vi "MainConvertiMisure_INPUT.vi"(6 "SET Q A ZERO":T1, 8 "canale--sensore":string[][](array[string]), 9 "Assoc_input_sensori":string[][](array[string]), 10 "Array Misure Input":dbl[](array[numeric]), 11 "Caratteristiche canali Caricate":string[][](array[string])) -> (2 "Array Misure/Unità OUT":T2[](array[typedef]))   [LabVIEW 2019]
uses:
  <vilib>/Analysis/6fits.llb/Curve Fitting Criteria.ctl
  <vilib>/Analysis/polynomials.llb/Scalar Polynomial Evaluation (DBL).vi
  <vilib>/Analysis/NI_AALPro.lvlib
  <vilib>/gmath/NI_Gmath.lvlib
panel:
  in  "Cluster Misura / Unità":T2
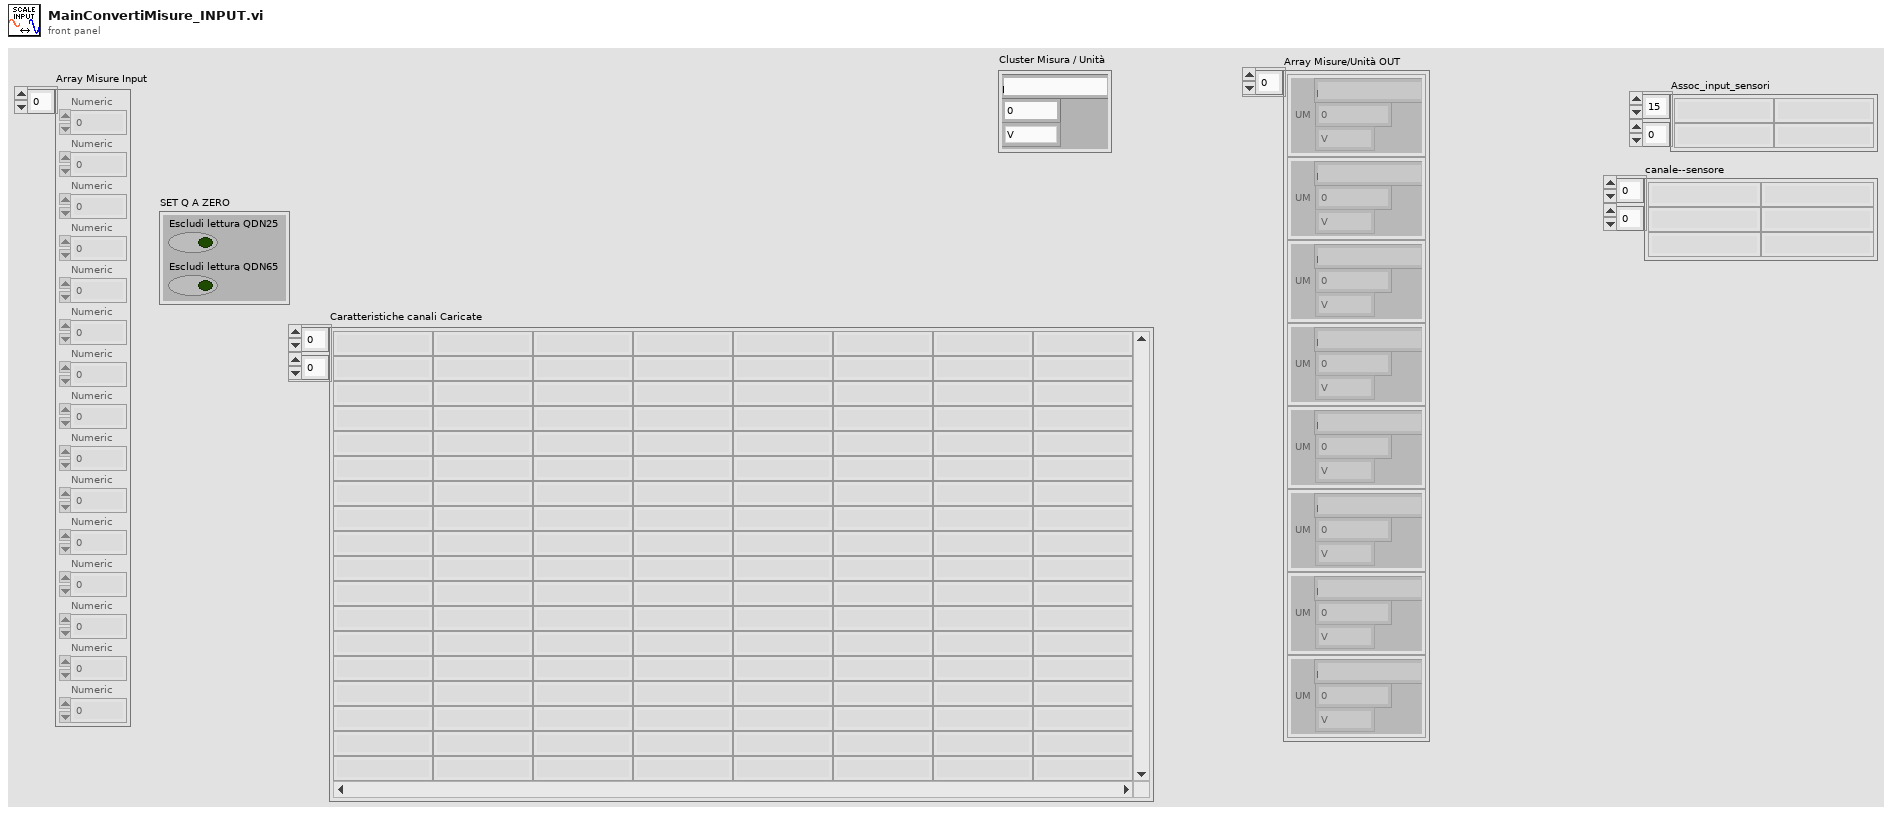
[diagram p1: front panel]
types:
  T1 = cluster{"Escludi lettura QDN25":bool, "Escludi lettura QDN65":bool}
  T2 = typedef "ClusterMisura_e_Unità_INPUT.ctl" = cluster{"Misura":dbl, "UM":T3, "Descrizione":string}
  T3 = typedef "UnitàMisura.ctl" = enum16{"V", "mA", "Bar", "RPM", "m3/s", "m3/min", "m3/h", "l/s", "l/min", "in3/min", "ft3/min", "gpm", "igpm", "igph", "%", "°C", "m", "Nm", "A"}
  T4 = cluster{"impostazioni conversione":string[], "um":i32}
  T5 = cluster{"ordine polinomiale":i32, "X":dbl[], "Y":dbl[]}
  T6 = typedef "NI_AALPro.lvlib/Curve Fitting Criteria.ctl" = u16
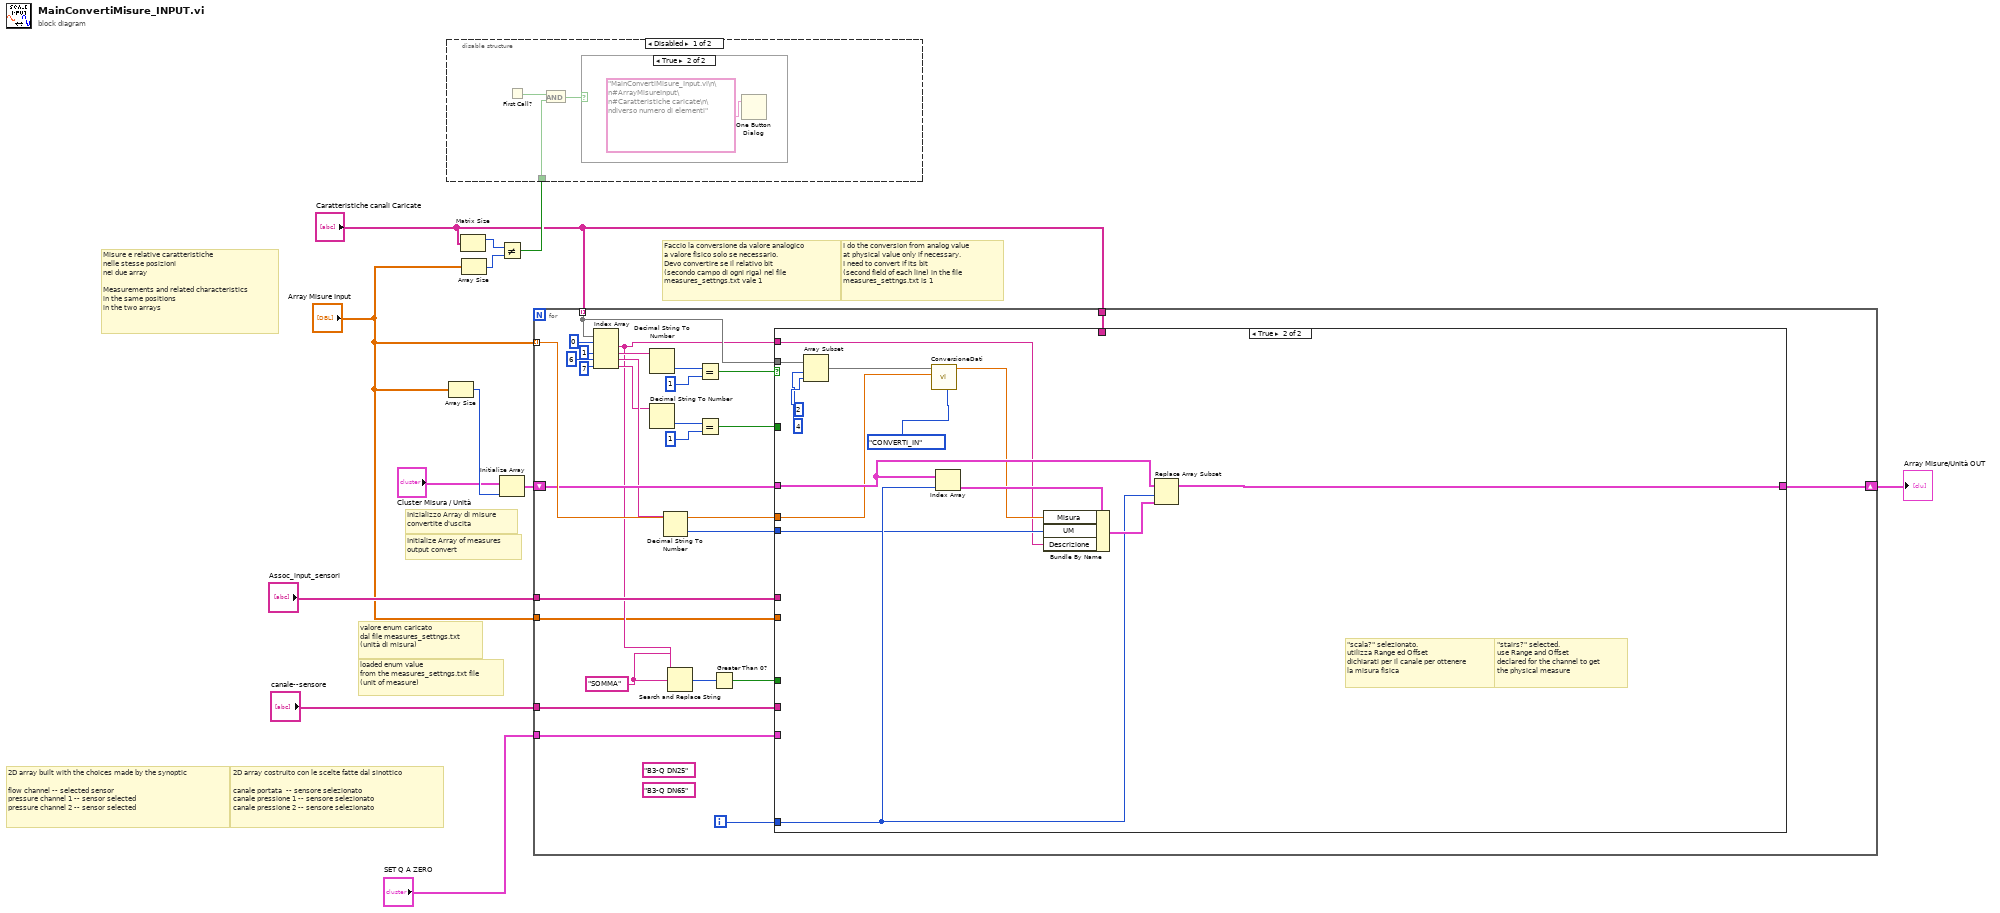
[diagram p0: block diagram]
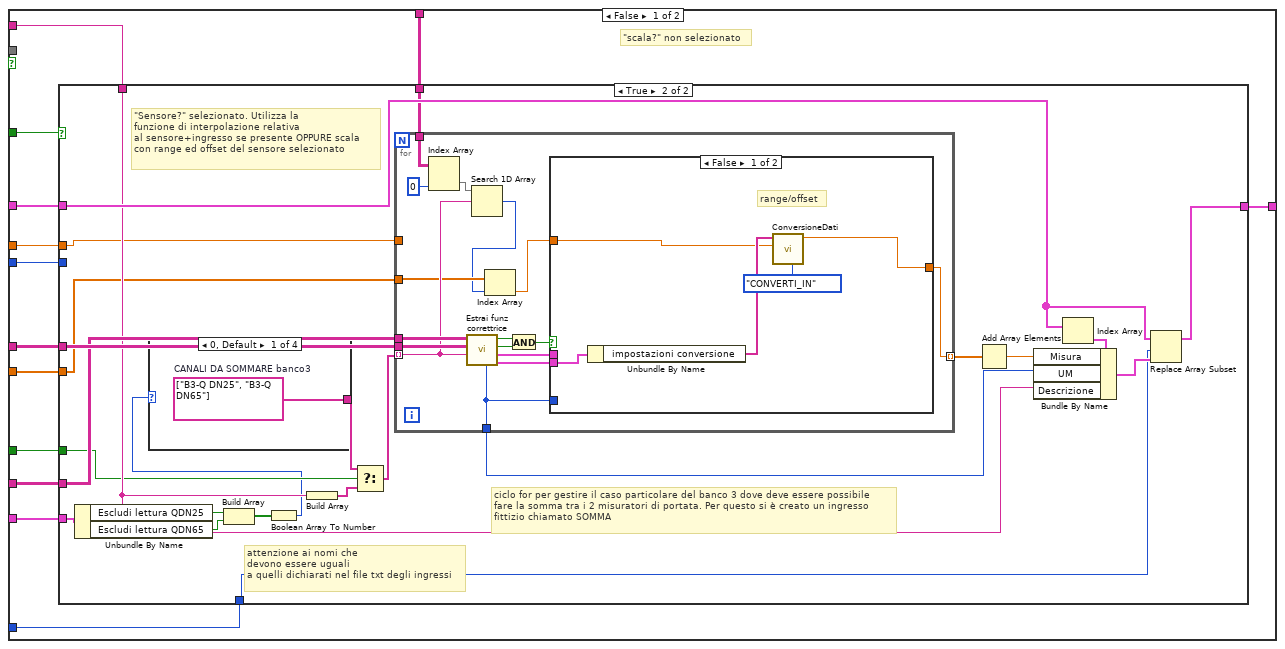
[diagram p4: hidden frame]
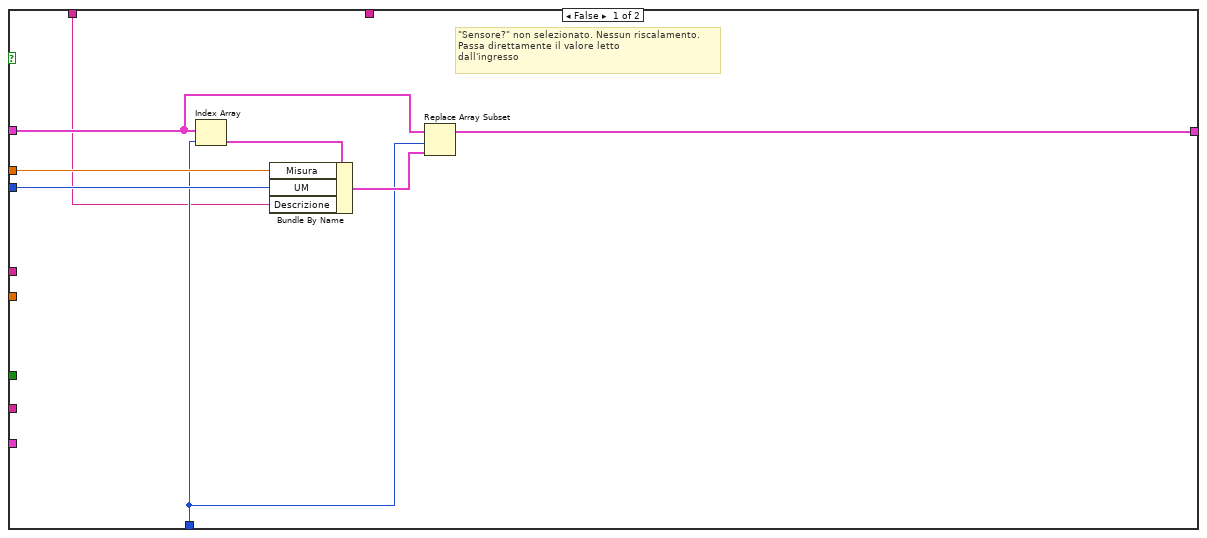
[diagram p5: hidden frame]
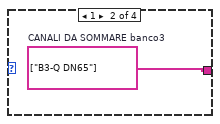
[diagram p6: hidden frame]
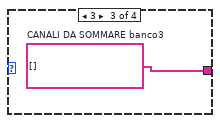
[diagram p7: hidden frame]
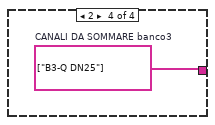
[diagram p8: hidden frame]
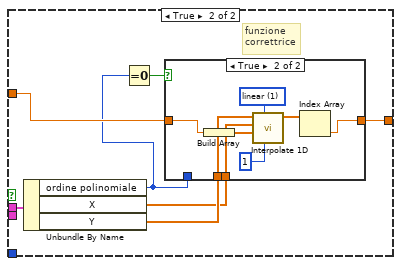
[diagram p9: hidden frame]
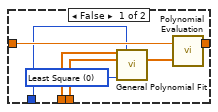
[diagram p10: hidden frame]
diagram:
  # "valore enum caricato\ndal file measures_settngs.txt \n(unità di misura)"
  # "loaded enum value\nfrom the measures_settngs.txt file\n(unit of measure)"
  # "Initialize Array of measures\noutput convert"
  # "2D array built with the choices made by the synoptic\n\nflow channel -- selected sensor\npressure channel 1 -- sensor selected\npressure channel 2 -- sensor selected"
  # "I do the conversion from analog value\nat physical value only if necessary.\nI need to convert if its bit\n(second field of each line) in the file\nmeasures_settngs.txt is 1"
  # "2D array costruito con le scelte fatte dal sinottico\n\ncanale portata  -- sensore selezionato\ncanale pressione 1 -- sensore selezionato\ncanale pressione 2 -- sensore selezionato"
  # "Faccio la conversione da valore analogico\na valore fisico solo se necessario. \nDevo convertire se il relativo bit \n(secondo campo di ogni riga) nel file \nmeasures_settngs.txt vale 1"
  # "Misure e relative caratteristiche\nnelle stesse posizioni\nnei due array\n\nMeasurements and related characteristics\nin the same positions\nin the two arrays"
  # "Inizializzo Array di misure \nconvertite d'uscita"
  n1 = Array Size(array="Array Misure Input") -> (size(s)=w12:i32)
  n2 = Matrix Size(0:"Caratteristiche canali Caricate") -> (1:w8:i32)  [unwired: 1 out]
  n3 = Array Size(array="Array Misure Input") -> (size(s)=w7:i32)
  n4 = Not Equal?(x=w8, y=w7) -> (x != y?=w6:bool)
  n5 = disable-structure shown="Disabled" {
    disable-tunnel: w6 -> [w14 _]
    frame Disabled {
      n6 = First Call?() -> (First Call?: T/F=w15:bool)
      n7 = And(x=w15, y=w14) -> (x .and. y?=w13:bool)
      n8 = case shown="True" w13 {
        frame False {
        }
        frame True {
          n9 = One Button Dialog(message="MainConvertiMisure_Input.vi\n\n#ArrayMisureInput\n#Caratteristiche caricate\n\ndiverso numero di elementi") -> ()  [unwired: 1 in, 1 out]
        }
      }
    }
    frame Enabled {
    }
  }
  n10 = Initialize Array("Cluster Misura / Unità", w12) -> (w11:T2[])
  n11 = for {
    tunnel: "Array Misure Input" -> [w39] mode=indexing
    tunnel: "Caratteristiche canali Caricate" -> [w33] mode=indexing
    shift-right: [w34] -> w9
    shift-left: w11 -> [w38]
    tunnel: "Assoc_input_sensori" -> [w25]
    tunnel: "canale--sensore" -> [w24]
    tunnel: "Array Misure Input" -> [w19]
    tunnel: "Caratteristiche canali Caricate" -> [w18]
    tunnel: "SET Q A ZERO" -> [w17]
    i -> [w32]
    (unwired) "B3-Q DN65"
    (unwired) "B3-Q DN25"
    w23 = "SOMMA" ("search string")
    n12 = Index Array(array=w33, index #1=0 ("index"), index #2=1 ("index"), index #3=6 ("index"), index #4=7 ("index")) -> (element #1=w21:string, element #2=w43:string, element #3=w36:string, element #4=w27:string)
    n13 = Decimal String To Number(string=w43) -> (number=w42:i32)  [unwired: 2 in, 1 out]
    n14 = Decimal String To Number(string=w27) -> (number=w28:i32)  [unwired: 2 in, 1 out]
    n15 = Decimal String To Number(string=w36) -> (number=w35:i32)  [unwired: 2 in, 1 out]
    n16 = Search and Replace String(input string=w21, search string=w23, replace string=w23) -> (number of replacements=w22:i32)  [unwired: 5 in, 3 out]
    n17 = Equal?(x=w42, y=1) -> (x = y?=w40:bool)
    n18 = Equal?(x=w28, y=1) -> (x = y?=w26:bool)
    n19 = Greater Than 0?(x=w22) -> (x > 0?=w20:bool)
    n20 = case shown="True" w40 {
      tunnel: w39 -> [w57 w141]
      tunnel: w38 -> [w55 w146]
      tunnel: w32 -> [w54 w148]
      tunnel: w35 -> [w56 w144]
      tunnel: [w53 w145] -> w34
      tunnel: w33 -> [_ w143]
      tunnel: w21 -> [w49 w136]
      tunnel: w26 -> [w52 _]
      tunnel: w25 -> [w51 _]
      tunnel: w24 -> [w50 _]
      tunnel: w20 -> [w48 _]
      tunnel: w19 -> [w47 _]
      tunnel: w18 -> [w46 _]
      tunnel: w17 -> [w45 _]
      frame False {
        # "\"scala?\" non selezionato"
        n21 = case shown="True" w52 {
          tunnel: w57 -> [w64 w78]
          tunnel: w56 -> [w63 _]
          tunnel: w55 -> [w61 w83]
          tunnel: w54 -> [w60 w84]
          tunnel: [w59 w82] -> w53
          tunnel: w49 -> [w58 w80]
          tunnel: w51 -> [_ w88]
          tunnel: w50 -> [_ w87]
          tunnel: w48 -> [_ w73]
          tunnel: w47 -> [_ w72]
          tunnel: w46 -> [_ w71]
          tunnel: w45 -> [_ w70]
          frame False {
            # "\"Sensore?\" non selezionato. Nessun riscalamento.\nPassa direttamente il valore letto\ndall'ingresso"
            n22 = Index Array(array=w61, index=w60) -> (element=w65:T2)
            n23 = Bundle By Name(cluster=w65, "Misura"=w64, "UM"=w63, "Descrizione"=w58) -> (w62:T2)
            n24 = Replace Array Subset(array=w61, new element=w62, index=w60) -> (w59:T2[])
          }
          frame True {
            # "ciclo for per gestire il caso particolare del banco 3 dove deve essere possibile\nfare la somma tra i 2 misuratori di portata. Per questo si è creato un ingresso\nfittizio chiamato SOMMA"
            # "attenzione ai nomi che \ndevono essere uguali\na quelli dichiarati nel file txt degli ingressi"
            # "\"Sensore?\" selezionato. Utilizza la\nfunzione di interpolazione relativa\nal sensore+ingresso se presente OPPURE scala \ncon range ed offset del sensore selezionato"
            n25 = Unbundle By Name(w70) -> ("Escludi lettura QDN25"=w69:bool, "Escludi lettura QDN65"=w68:bool)
            n26 = Build Array(w69, w68) -> (w67:bool[])
            n27 = Boolean Array To Number(Boolean array=w67) -> (number=w66:u32)
            n28 = case shown="0, Default" w66 {
              tunnel: [w89 w90 w91 w92] -> w76
              frame 0, Default {
                w89 = string[] ["B3-Q DN25", "B3-Q DN65"]  # CANALI DA SOMMARE banco3
              }
              frame 1 {
                w90 = string[] ["B3-Q DN65"]  # CANALI DA SOMMARE banco3
              }
              frame 3 {
                w91 = string[] []  # CANALI DA SOMMARE banco3
              }
              frame 2 {
                w92 = string[] ["B3-Q DN25"]  # CANALI DA SOMMARE banco3
              }
            }
            n29 = Build Array(w80) -> (w75:string[])
            n30 = Select(t=w76, s=w73, f=w75) -> (s? t:f=w74:string[])
            n31 = for {
              tunnel: w88 -> [w108]
              tunnel: w87 -> [w107]
              tunnel: [w101] -> w81
              tunnel: [w100] -> w79 mode=indexing
              tunnel: w78 -> [_]
              tunnel: w74 -> [w96] mode=indexing
              tunnel: w72 -> [w95]
              tunnel: w71 -> [w99]
              n32 = Index Array(array=w99, index (col)=0 ("disabled index (col)")) -> (element=w97:string[])  [unwired: 1 in]
              n33 = call "Estrai funz correttrice.vi"("nome canale"=w96, "Assoc_input_sensori"=w108, "canale--sensore"=w107) -> ("conv. con range offset"=w104:T4, "INTERPOLAZIONE SETTINGS"=w105:T5, "USA FUNZ CORR"=w102:bool, "FUNZ CORR PRESENTE"=w103:bool, "um"=w101:i32)  [unwired: 4 in]
              n34 = Search 1D Array(1D array=w97, element=w96) -> (index of element=w94:i32)  [unwired: 1 in]
              n35 = Index Array(array=w95, index=w94) -> (element=w93:dbl)
              n36 = And(x=w103, y=w102) -> (x .and. y?=w106:bool)
              n37 = case shown="False" w106 {
                tunnel: w105 -> [_ w120]
                tunnel: w93 -> [w110 w117]
                tunnel: w104 -> [w112 _]
                tunnel: w101 -> [_ _]
                tunnel: [w109 w116] -> w100
                frame False {
                  # "range/offset"
                  n38 = Unbundle By Name(w112) -> ("impostazioni conversione"=w111:string[])
                  n39 = call "ConversioneDati.vi"("Stato Conversione"=enum16{"CONVERTI_IN", "CONVERTI_OUT"}."CONVERTI_IN", "Data"=w110, "Impostazioni Conversione"=w111) -> ("Dato Convertito"=w109:dbl)  [unwired: 8 in]
                }
                frame True {
                  # "funzione\ncorrettrice"
                  n40 = Unbundle By Name(w120) -> ("ordine polinomiale"=w114:i32, "X"=w118:dbl[], "Y"=w119:dbl[])
                  n41 = Equal To 0?(x=w114) -> (x = 0?=w115:bool)
                  n42 = case shown="True" w115 {
                    tunnel: w119 -> [w126 w134]
                    tunnel: w118 -> [w125 w135]
                    tunnel: w117 -> [w123 w129]
                    tunnel: [w122 w130] -> w116
                    tunnel: w114 -> [w121 _]
                    frame False {
                      w127 = T6 0 items=["Least Square", "Least Absolute Residual", "Bisquare"] ("method")
                      n43 = call <vilib>:"General Polynomial Fit.vi"("Y"=w126, "polynomial order"=w121, "X"=w125, "method"=w127) -> ("Polynomial Coefficients"=w124:dbl[])  [unwired: 8 in, 3 out]
                      n44 = call-poly <vilib>:"Polynomial Evaluation.vi"("P(x)"=w124, "a"=w123) -> ("P(a)"=w122:dbl)  [unwired: 1 out]
                    }
                    frame True {
                      w133 = 1 items=["nearest", "linear", "spline", "cubic Hermite", "Lagrange"] ("method")
                      n45 = Build Array(w129) -> (w128:dbl[])
                      n46 = call <vilib>:"Interpolate 1D.vi"("ntimes"=1, "method"=w133, "xi"=w128, "X"=w135, "Y"=w134) -> ("yi"=w131:dbl[])  [unwired: 4 in, 2 out]
                      n47 = Index Array(array=w131) -> (element=w130:dbl)  [unwired: 1 in]
                    }
                  }
                }
              }
            }
            n48 = Add Array Elements(numeric array=w79) -> (sum=w77:dbl)
            n49 = Index Array(array=w83) -> (element=w86:T2)  [unwired: 1 in]
            n50 = Bundle By Name(cluster=w86, "Misura"=w77, "UM"=w81, "Descrizione"=w80) -> (w85:T2)
            n51 = Replace Array Subset(array=w83, new element=w85, index=w84) -> (w82:T2[])
          }
        }
      }
      frame True {
        # "\"stairs?\" selected.\nuse Range and Offset\ndeclared for the channel to get\nthe physical measure"
        # "\"scala?\" selezionato.\nutilizza Range ed Offset\ndichiarati per il canale per ottenere\nla misura fisica"
        n52 = Array Subset(array=w143, index=2, length=4 ("index")) -> (w142:string[])
        n53 = call "ConversioneDati.vi"("Stato Conversione"=enum16{"CONVERTI_IN", "CONVERTI_OUT"}."CONVERTI_IN", "Data"=w141, "Impostazioni Conversione"=w142) -> ("Dato Convertito"=w140:dbl)  [unwired: 8 in]
        n54 = Index Array(array=w146, index=w148) -> (element=w147:T2)
        n55 = Bundle By Name(cluster=w147, "Misura"=w140, "UM"=w144, "Descrizione"=w136) -> (w149:T2)
        n56 = Replace Array Subset(array=w146, new element=w149, index=w148) -> (w145:T2[])
      }
    }
  }
  "Array Misure/Unità OUT" <- w9
